vi "ExecuteOrRecurse.vi"(6 "Error":errorcluster, 10 "Message":refnum<class "Message.lvclass">, 11 "Actor":refnum<class "Actor.lvclass">) -> (2 "Message":refnum<class "Message.lvclass">, 3 "Actor":refnum<class "Actor.lvclass">, 4 "Error":errorcluster)   [LabVIEW 2020, in "jettl.lvlib"]
uses:
  jettl.lvlib
  Actor/Actor.lvclass
  Message/Message.lvclass
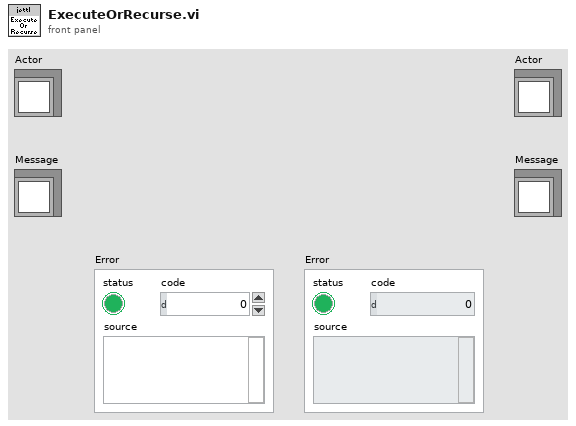
[diagram p1: front panel]
types:
  T1 = typedef "jettl.lvlib/BaseActor.ctl" = cluster{"Lifetime":T2, "SelfActor":T3, "MediatorActor":T3, "ComponentActorMap":T8}
  T2 = typedef "jettl.lvlib/Lifetime.ctl" = enum16{"Init", "Spawn", "Setup", "TeardownBeforeRunning", "Running", "StopCalled", "StoppingWithComponents", "StoppingNoComponents", "TeardownAfterRunning", "Stopped"}
  T3 = typedef "jettl.lvlib/Actor.ctl" = cluster{"Messages":T4, "ActorAlias":string, "ActorType":T7, "Transport":refnum<user-event>, "VIRef":refnum<vi>}
  T4 = typedef "jettl.lvlib/Messages.ctl" = cluster{"Listen":T5, "TellSelf":T5, "TellMediator":T5, "TellComponentMap":T6}
  T5 = typedef "jettl.lvlib/MessageSet.ctl" = set{refnum<class "Message.lvclass">}
  T6 = typedef "jettl.lvlib/TellComponentMap.ctl" = map{string, T5}
  T7 = typedef "jettl.lvlib/ActorType.ctl" = enum16{"Mediator", "Component"}
  T8 = typedef "jettl.lvlib/ComponentActorMap.ctl" = map{string, T3}
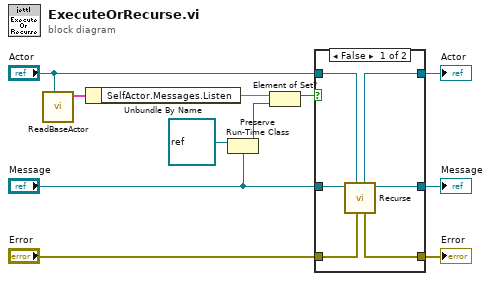
[diagram p0: block diagram]
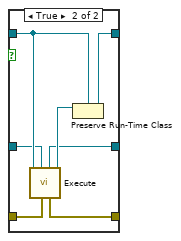
[diagram p2: hidden frame]
diagram:
  n1 = call-dynamic "ReadBaseActor.vi"("Actor"="Actor") -> ("BaseActor"=w7:T1)  [unwired: 10 in]
  n2 = Unbundle By Name(w7) -> ("SelfActor.Messages.Listen"=w6:T5)
  n3 = Preserve Run-Time Class(object in=refnum<class> refnum, 2:"Message") -> (object out=w1:refnum<class "Message.lvclass">)  [unwired: 1 in, 1 out]
  n4 = Element of Set?(10:w1, 11:w6) -> (3:w5:bool)
  n5 = case shown="False" w5 {
    tunnel: "Actor" -> [w17 w24]
    tunnel: [w16 w20] -> w10
    tunnel: [w14 w22] -> w11
    tunnel: "Error" -> [w15 w23]
    tunnel: "Message" -> [w13 w21]
    tunnel: [w12 w18] -> w4
    frame False {
      n6 = call-dynamic "Recurse.vi"("Error"=w15, "Actor"=w17, "Message"=w13) -> ("Message"=w12:refnum<class "Message.lvclass">, "Error"=w14:errorcluster, "Actor"=w16:refnum<class "Actor.lvclass">)  [unwired: 6 in]
    }
    frame True {
      n7 = call-dynamic "Execute.vi"("Error"=w23, "Message"=w21, "Actor"=w24) -> ("Actor"=w19:refnum<class "Actor.lvclass">, "Error"=w22:errorcluster, "Message"=w18:refnum<class "Message.lvclass">)  [unwired: 6 in]
      n8 = Preserve Run-Time Class(object in=w19, 2:w24) -> (object out=w20:refnum<class "Actor.lvclass">)  [unwired: 1 in, 1 out]
    }
  }
  "Error" <- w11
  "Actor" <- w10
  "Message" <- w4
